vi "Motor Controller Get and clear error state byte.vi"(10 "RS-485 addr.":u8=1 min=1, 11 "COM port":refnum<visa-resource-name>) -> (0 "Error out":errorcluster, 1 "Checksum ok":bool, 2 "Frame ok":bool, 3 "Error bits":bool[](array[boolean]))   [LabVIEW 2020]
uses:
  ctls/CTRL_Cmd.ctl
panel:
  # "EEPROM bad checksum\n\nUSB data bad frame\n\nUSB data bad checksum 1\n\nUSB data bad checksum 2\n\nRS-485 data bad frame\n\nRS-485 data bad checksum 1\n\nRS-485 data bad checksum 2"
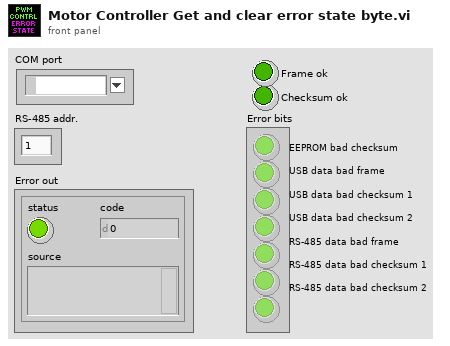
[diagram p1: front panel]
types:
  T1 = typedef "CTRL_Cmd.ctl" = string
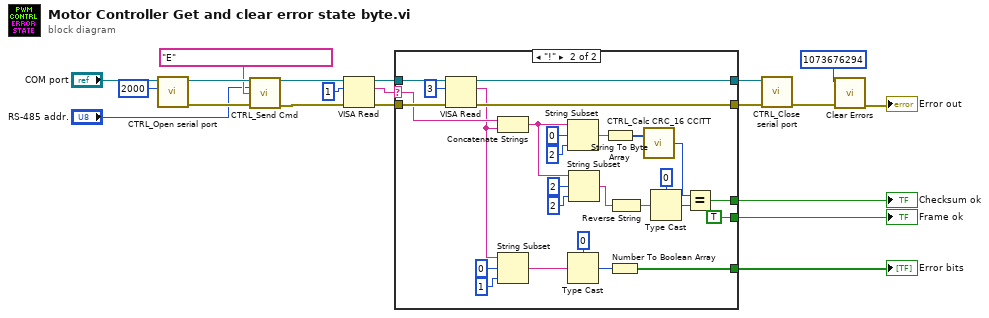
[diagram p0: block diagram]
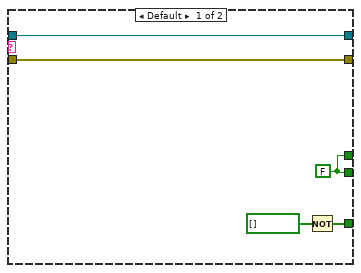
[diagram p2: hidden frame]
diagram:
  n1 = call "CTRL_Open serial port.vi"("timeout (ms)"=u32 2000, "VISA resource name"="COM port") -> ("Error out"=w10:errorcluster, "VISA resource name out"=w17:refnum<visa-resource-name>)  [unwired: 8 in]
  n2 = call "CTRL_Send Cmd.vi"("Port"=w17, "RS-485 addr."="RS-485 addr.", "Cmd"=T1 "E" ("Command"), "Error In"=w10) -> ("Port out"=w18:refnum<visa-resource-name>, "Error Out"=w19:errorcluster)  [unwired: 10 in]
  n3 = VISA Read(VISA resource name=w18, byte count=u32 1, error in (no error)=w19) -> (VISA resource name out=w13:refnum<visa-resource-name>, read buffer=w12:string, error out=w14:errorcluster)  [unwired: 1 out]
  n4 = case shown="\"!\"" w12 {
    selector: w12 -> [_ w47]
    tunnel: w14 -> [w25 w51]
    tunnel: w13 -> [w24 w52]
    tunnel: [w25 w49] -> w5
    tunnel: [w24 w48] -> w4
    tunnel: [w23 w34] -> w9
    tunnel: [w23 TRUE] -> w8
    tunnel: [w21 w26] -> w6
    frame Default {
      w23 = FALSE
      n5 = Not(x=bool[] [] ("Boolean array")) -> (.not. x?=w21:bool[])
    }
    frame "!" {
      n6 = VISA Read(VISA resource name=w52, byte count=u32 3, error in (no error)=w51) -> (VISA resource name out=w48:refnum<visa-resource-name>, read buffer=w32:string, error out=w49:errorcluster)  [unwired: 1 out]
      n7 = Concatenate Strings(w47, w32) -> (w33:string)
      n8 = String Subset(string=w32, offset (0)=0, length (rest)=1 ("length (rest)")) -> (substring=w29:string)
      n9 = String Subset(string=w33, offset (0)=0, length (rest)=2 ("length (rest)")) -> (substring=w36:string)
      n10 = Type Cast(type=u8 0, x=w29) -> (*(type *) &x=w27:u8)
      n11 = String Subset(string=w33, offset (0)=2, length (rest)=2 ("length (rest)")) -> (substring=w43:string)
      n12 = String To Byte Array(string=w36) -> (unsigned byte array=w46:u8[])
      n13 = Number To Boolean Array(number=w27) -> (Boolean array=w26:bool[])
      n14 = Reverse String(1:w43) -> (0:w41:string)
      n15 = call "CTRL_Calc CRC_16 CCITT.vi"("Data bytes"=w46) -> ("CRC_16-CCITT"=w40:u16)  [unwired: 1 in]
      n16 = Type Cast(type=u16 0 ("length (rest)"), x=w41) -> (*(type *) &x=w39:u16)
      n17 = Equal?(x=w40, y=w39) -> (x = y?=w34:bool)
    }
  }
  "Checksum ok" <- w9
  "Frame ok" <- w8
  "Error bits" <- w6
  n18 = call "CTRL_Close serial port.vi"("Error in"=w5, "VISA resource name"=w4) -> ("Error out"=w2:errorcluster)  [unwired: 9 in]
  n19 = call <vilib>:"Clear Errors.vi"("error in (no error)"=w2, "specific error code to clear (0: all)"=1073676294) -> ("error out"=→"Error out":errorcluster)  [unwired: 4 in, 1 out]
